vi "LVDimInterface.dim_fire_occurrence.vi"(5 "error in (no error)":errorcluster) -> (19 "error out":errorcluster)   [LabVIEW 2015, in "LVDimInterface.lvlib"]
doc: "This routine can be called by a server or a client program to programmatically fire (set) the occurrence that has previously been registered using the routine dim_set_occurrence_ref. \n\nHistory: 24-OCT-2007, Dietrich Beck\n\nCopyright (C)\nGesellschaft für Schwerionenforschung, GSI\nPlanckstr. 1\n64291 Darmstadt\nGermany\n\nContact: D.Beck@gsi.de \n\nThis program is free software; you can redistribute it and/or modify it under the terms of the \nGNU General Public License as published by the Free Software Foundation; either version 2 of the license, or (at your option) any later version.\n\nThis program is distributed in the hope that it will be useful, but WITHOUT ANY WARRANTY; without even the implied warranty of MERCHANTABILITY or FITNESS FOR A PARTICULAR PURPOSE. See the GNU General License for more details (http://www.gnu.org).\n\nGesellschaft für Schwerionenforschung, GSI\nPlanckstr. 1, 64291 Darmstadt, Germany\nFor all questions and ideas contact D. Beck.\nLast update: 16-DEC-2005"
uses:
  LVDimInterface.lvlib
  bin/libDimWrapper.dll
  bin/libDimWrapper.so
  bin/libDimWrapperSPL.dll
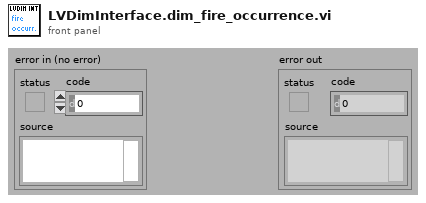
[diagram p1: front panel]
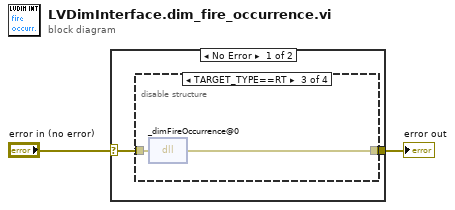
[diagram p0: block diagram]
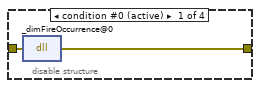
[diagram p2: hidden frame]
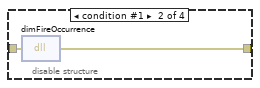
[diagram p3: hidden frame]
diagram:
  n1 = case shown="No Error" "error in (no error)" {
    selector: "error in (no error)" -> [w4 w12]
    tunnel: [w3 w12] -> w2
    frame No Error {
      n2 = disable-structure "Conditional Disable Structure" shown="TARGET_TYPE==RT" {
        disable-tunnel: w4 -> [w6 w7 w10 w11]
        disable-tunnel: [w5 w8 w9 w11] -> w3
        frame condition #0 (active) {
          n3 = dll-call lib="D:/Git/CSPP/Packages/DimLVEvent/bin/libDimWrapper.dll" fn="_dimFireOccurrence@0"(error in=w6) -> (error out=w5:errorcluster)  [unwired: 3 in, 1 out]
        }
        frame condition #1 {
          n4 = dll-call lib="D:/Git/CS-framework/CSlibraries/DimLVEvent/bin/libDimWrapper.so" fn="dimFireOccurrence" label="libDimWrapper.dll:_dimFireOccurrence@0"(error in=w7) -> (error out=w8:errorcluster)  [unwired: 3 in, 1 out]
        }
        frame condition #2 {
          n5 = dll-call lib="D:/Git/CS-framework/CSlibraries/DimLVEvent/bin/libDimWrapperSPL.dll" fn="_dimFireOccurrence@0"(error in=w10) -> (error out=w9:errorcluster)  [unwired: 3 in, 1 out]
        }
        frame condition #3 {
        }
      }
    }
    frame Error {
    }
  }
  "error out" <- w2
